vi "AddStartEndPointsGrid.vi"(4 "Xgoal":dbl format="%#_13g", 5 "Xstart":dbl format="%#_13g", 6 "GridParameter":dbl, 7 "Ystart":dbl format="%#_13g", 8 "n vertical":dbl, 9 "Ygoal":dbl format="%#_13g", 10 "n horizontal":dbl, 11 "grid in":T1) -> (0 "Nó goal":dbl[](array[numeric]), 1 "Nó start":dbl[](array[numeric]), 2 "grid out":T1)   [LabVIEW 2016]
uses:
  grid.ctl
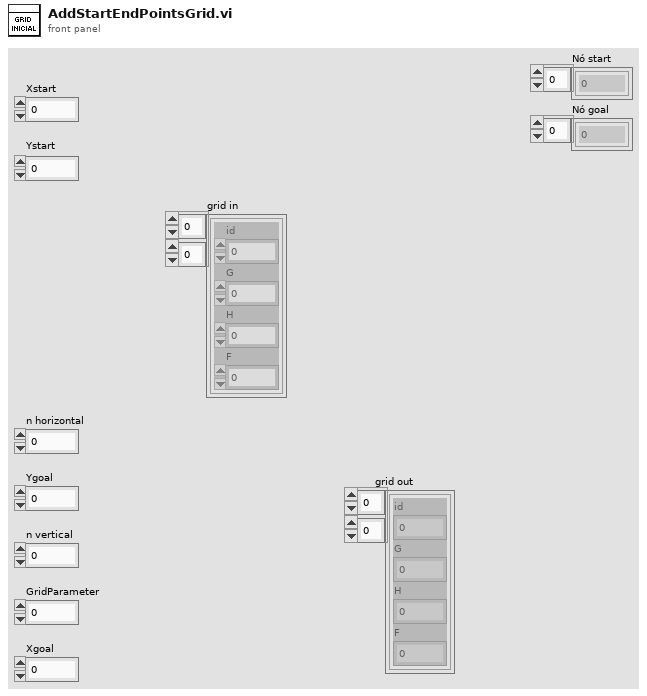
[diagram p1: front panel]
types:
  T1 = typedef "grid.ctl" = cluster{"id":dbl, "G":dbl, "H":dbl, "F":dbl}[][]
  T2 = cluster{"[0]":dbl, "[1]":dbl, "[2]":dbl, "[3]":dbl}
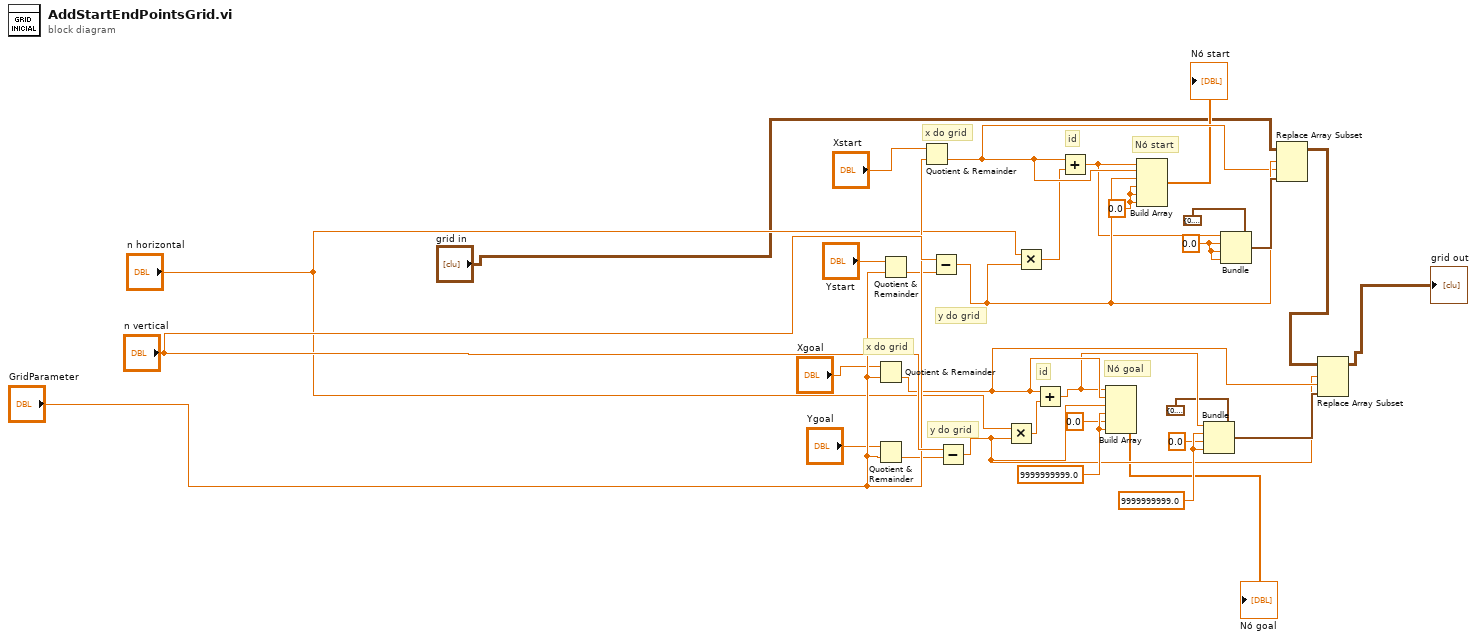
[diagram p0: block diagram]
diagram:
  w29 = 9999999999.0
  w28 = 9999999999.0
  w17 = 0.0 ("element")
  w15 = 0.0 ("element")
  # "Nó goal"
  # "Nó start"
  # "id"
  # "y do grid"
  # "x do grid"
  # "id"
  # "y do grid"
  # "x do grid"
  n1 = Quotient & Remainder(x="Xgoal", y="GridParameter") -> (floor(x/y)=w26:dbl)  [unwired: 1 out]
  n2 = Quotient & Remainder(x="Ygoal", y="GridParameter") -> (floor(x/y)=w12:dbl)  [unwired: 1 out]
  n3 = Quotient & Remainder(x="Ystart", y="GridParameter") -> (floor(x/y)=w8:dbl)  [unwired: 1 out]
  n4 = Quotient & Remainder(x="Xstart", y="GridParameter") -> (floor(x/y)=w22:dbl)  [unwired: 1 out]
  n5 = Subtract(x="n vertical", y=w8) -> (x-y=w23:dbl)
  n6 = Subtract(x="n vertical", y=w12) -> (x-y=w25:dbl)
  n7 = Multiply(x="n horizontal", y=w25) -> (x*y=w13:dbl)
  n8 = Multiply(x="n horizontal", y=w23) -> (x*y=w9:dbl)
  n9 = Add(x=w26, y=w13) -> (x+y=w20:dbl)
  n10 = Add(x=w22, y=w9) -> (x+y=w16:dbl)
  n11 = Build Array(w20, w26, w25, w29, 0.0 ("element"), w29) -> (→"Nó goal":dbl[])
  n12 = Build Array(w16, w22, w23, w15, w15, w15) -> (→"Nó start":dbl[])
  n13 = Bundle(cluster=T2 {"[0]"=0.0, "[1]"=0.0, "[2]"=0.0, "[3]"=0.0} ("element 2"), "[0]"=w20, "[1]"=w28, "[2]"=0.0 ("element"), "[3]"=w28) -> (w27:T2)
  n14 = Bundle(cluster=T2 {"[0]"=0.0, "[1]"=0.0, "[2]"=0.0, "[3]"=0.0} ("element 2"), "[0]"=w16, "[1]"=w17, "[2]"=w17, "[3]"=w17) -> (w24:T2)
  n15 = Replace Array Subset(array="grid in", new element=w24, index (row)=w23, index (col)=w22) -> (w19:T1)
  n16 = Replace Array Subset(array=w19, new element=w27, index (row)=w25, index (col)=w26) -> (→"grid out":T1)
